vi "Hardware-ESTTL-Host.vi"() -> ()   [LabVIEW 2016]
uses:
  <vilib>/Powertrain Controls/Device Drivers/DCM/ESTTL/RT/Setup.ctl
  <vilib>/Powertrain Controls/Device Drivers/DCM/ESTTL/FPGA/Mode.ctl
  <vilib>/Powertrain Controls/Device Drivers/DCM/ESTTL/RT/Angle Control.ctl
  Shared/Typedefs/DiffIO-PWM-Settings.ctl
  Shared/Typedefs/DiffIO-PWM-Settings-Array.ctl
  Shared/DSI-Shared.lvlib
  <vilib>/Powertrain Controls/Device Drivers/DCM/ESTTL/FPGA/DCM - FPGA - ESTTL.lvlib
  <vilib>/Powertrain Controls/Device Drivers/DCM/ESTTL/RT/DCM - RT - ESTTL.lvlib
panel:
  in  "_Hidden":enum32{"Page 1"}(tab)
  in  "Setup":T1[](array[typedef])=[{"Mode"=enum."Off", "Polarity"=FALSE, "Frequency [Hz]"=0.0, "Duty Cycle [%]"=0.0, "TDC Offset [CAD]"=0.0, "Window Start [DBTDC]"=0.0, "Window End [DBTDC]"=0.0, "Angles"=[{"Enable"=FALSE, "Location [DBTDC]"=0.0, "Duration [s]"=0.0}, {"Enable"=FALSE, "Location [DBTDC]"=0.0, "Duration [s]"=0.0}, {"Enable"=FALSE, "Location [DBTDC]"=0.0, "Duration [s]"=0.0}, {"Enable"=FALSE, "Location [DBTDC]"=0.0, "Duration [s]"=0.0}], "Skip Fire"=FALSE, "Skip Fire Index"=0}, {"Mode"=enum."Off", "Polarity"=FALSE, "Frequency [Hz]"=0.0, "Duty Cycle [%]"=0.0, "TDC Offset [CAD]"=0.0, "Window Start [DBTDC]"=0.0, "Window End [DBTDC]"=0.0, "Angles"=[{"Enable"=FALSE, "Location [DBTDC]"=0.0, "Duration [s]"=0.0}, {"Enable"=FALSE, "Location [DBTDC]"=0.0, "Duration [s]"=0.0}, {"Enable"=FALSE, "Location [DBTDC]"=0.0, "Duration [s]"=0.0}, {"Enable"=FALSE, "Location [DBTDC]"=0.0, "Duration [s]"=0.0}], "Skip Fire"=FALSE, "Skip Fire Index"=0}, {"Mode"=enum."Off", "Polarity"=FALSE, "Frequency [Hz]"=0.0, "Duty Cycle [%]"=0.0, "TDC Offset [CAD]"=0.0, "Window Start [DBTDC]"=0.0, "Window End [DBTDC]"=0.0, "Angles"=[{"Enable"=FALSE, "Location [DBTDC]"=0.0, "Duration [s]"=0.0}, {"Enable"=FALSE, "Location [DBTDC]"=0.0, "Duration [s]"=0.0}, {"Enable"=FALSE, "Location [DBTDC]"=0.0, "Duration [s]"=0.0}, {"Enable"=FALSE, "Location [DBTDC]"=0.0, "Duration [s]"=0.0}], "Skip Fire"=FALSE, "Skip Fire Index"=0}, {"Mode"=enum."Off", "Polarity"=FALSE, "Frequency [Hz]"=0.0, "Duty Cycle [%]"=0.0, "TDC Offset [CAD]"=0.0, "Window Start [DBTDC]"=0.0, "Window End [DBTDC]"=0.0, "Angles"=[{"Enable"=FALSE, "Location [DBTDC]"=0.0, "Duration [s]"=0.0}, {"Enable"=FALSE, "Location [DBTDC]"=0.0, "Duration [s]"=0.0}, {"Enable"=FALSE, "Location [DBTDC]"=0.0, "Duration [s]"=0.0}, {"Enable"=FALSE, "Location [DBTDC]"=0.0, "Duration [s]"=0.0}], "Skip Fire"=FALSE, "Skip Fire Index"=0}, {"Mode"=enum."Off", "Polarity"=FALSE, "Frequency [Hz]"=0.0, "Duty Cycle [%]"=0.0, "TDC Offset [CAD]"=0.0, "Window Start [DBTDC]"=0.0, "Window End [DBTDC]"=0.0, "Angles"=[{"Enable"=FALSE, "Location [DBTDC]"=0.0, "Duration [s]"=0.0}, {"Enable"=FALSE, "Location [DBTDC]"=0.0, "Duration [s]"=0.0}, {"Enable"=FALSE, "Location [DBTDC]"=0.0, "Duration [s]"=0.0}, {"Enable"=FALSE, "Location [DBTDC]"=0.0, "Duration [s]"=0.0}], "Skip Fire"=FALSE, "Skip Fire Index"=0}, {"Mode"=enum."Off", "Polarity"=FALSE, "Frequency [Hz]"=0.0, "Duty Cycle [%]"=0.0, "TDC Offset [CAD]"=0.0, "Window Start [DBTDC]"=0.0, "Window End [DBTDC]"=0.0, "Angles"=[{"Enable"=FALSE, "Location [DBTDC]"=0.0, "Duration [s]"=0.0}, {"Enable"=FALSE, "Location [DBTDC]"=0.0, "Duration [s]"=0.0}, {"Enable"=FALSE, "Location [DBTDC]"=0.0, "Duration [s]"=0.0}, {"Enable"=FALSE, "Location [DBTDC]"=0.0, "Duration [s]"=0.0}], "Skip Fire"=FALSE, "Skip Fire Index"=0}, {"Mode"=enum."Off", "Polarity"=FALSE, "Frequency [Hz]"=0.0, "Duty Cycle [%]"=0.0, "TDC Offset [CAD]"=0.0, "Window Start [DBTDC]"=0.0, "Window End [DBTDC]"=0.0, "Angles"=[{"Enable"=FALSE, "Location [DBTDC]"=0.0, "Duration [s]"=0.0}, {"Enable"=FALSE, "Location [DBTDC]"=0.0, "Duration [s]"=0.0}, {"Enable"=FALSE, "Location [DBTDC]"=0.0, "Duration [s]"=0.0}, {"Enable"=FALSE, "Location [DBTDC]"=0.0, "Duration [s]"=0.0}], "Skip Fire"=FALSE, "Skip Fire Index"=0}, {"Mode"=enum."Off", "Polarity"=FALSE, "Frequency [Hz]"=0.0, "Duty Cycle [%]"=0.0, "TDC Offset [CAD]"=0.0, "Window Start [DBTDC]"=0.0, "Window End [DBTDC]"=0.0, "Angles"=[{"Enable"=FALSE, "Location [DBTDC]"=0.0, "Duration [s]"=0.0}, {"Enable"=FALSE, "Location [DBTDC]"=0.0, "Duration [s]"=0.0}, {"Enable"=FALSE, "Location [DBTDC]"=0.0, "Duration [s]"=0.0}, {"Enable"=FALSE, "Location [DBTDC]"=0.0, "Duration [s]"=0.0}], "Skip Fire"=FALSE, "Skip Fire Index"=0}] {"Skip Fire Index" max=7; "Angles"."Duration [s]" format="%#_3p"; "Frequency [Hz]" format="%#_3p"}
  in  "_Refresh":bool
  in  "AdaptMode":u32
  in  "ChannelNames":string[](array[string])
  in  "PWMSettings":T4=[{"PWM-TimingMode"=enum."Frequency", "PWM-Frequency"=0.0, "PWM-Period"=0.0, "PWM-ControlMode"=enum."Duty Cycle", "PWM-DutyCycle"=0.0, "PWM-PulseWidth"=0.0}, {"PWM-TimingMode"=enum."Frequency", "PWM-Frequency"=0.0, "PWM-Period"=0.0, "PWM-ControlMode"=enum."Duty Cycle", "PWM-DutyCycle"=0.0, "PWM-PulseWidth"=0.0}, {"PWM-TimingMode"=enum."Frequency", "PWM-Frequency"=0.0, "PWM-Period"=0.0, "PWM-ControlMode"=enum."Duty Cycle", "PWM-DutyCycle"=0.0, "PWM-PulseWidth"=0.0}, {"PWM-TimingMode"=enum."Frequency", "PWM-Frequency"=0.0, "PWM-Period"=0.0, "PWM-ControlMode"=enum."Duty Cycle", "PWM-DutyCycle"=0.0, "PWM-PulseWidth"=0.0}, {"PWM-TimingMode"=enum."Frequency", "PWM-Frequency"=0.0, "PWM-Period"=0.0, "PWM-ControlMode"=enum."Duty Cycle", "PWM-DutyCycle"=0.0, "PWM-PulseWidth"=0.0}, {"PWM-TimingMode"=enum."Frequency", "PWM-Frequency"=0.0, "PWM-Period"=0.0, "PWM-ControlMode"=enum."Duty Cycle", "PWM-DutyCycle"=0.0, "PWM-PulseWidth"=0.0}, {"PWM-TimingMode"=enum."Frequency", "PWM-Frequency"=0.0, "PWM-Period"=0.0, "PWM-ControlMode"=enum."Duty Cycle", "PWM-DutyCycle"=0.0, "PWM-PulseWidth"=0.0}, {"PWM-TimingMode"=enum."Frequency", "PWM-Frequency"=0.0, "PWM-Period"=0.0, "PWM-ControlMode"=enum."Duty Cycle", "PWM-DutyCycle"=0.0, "PWM-PulseWidth"=0.0}] caption="Advanced PWM Settings" {"PWM-Period" format="%#_2p"; "PWM-PulseWidth" format="%#_2p"; "PWM-DutyCycle" format="%#_2p"; "PWM-Frequency" format="%#_2p"}
  in  "_PWM Settings Element":T5 caption="Advanced PWM Settings" {"PWM-Period" format="%#_2p"; "PWM-PulseWidth" format="%#_2p"; "PWM-DutyCycle" format="%#_2p"; "PWM-Frequency" format="%#_2p"}
  in  "_Setup Tab":enum32{"Page 1"}(tab)
  in  "_SetupElement":T1={"Mode"=enum."Off", "Polarity"=FALSE, "Frequency [Hz]"=0.0, "Duty Cycle [%]"=0.0, "TDC Offset [CAD]"=0.0, "Window Start [DBTDC]"=0.0, "Window End [DBTDC]"=0.0, "Angles"=[{"Enable"=FALSE, "Location [DBTDC]"=0.0, "Duration [s]"=0.0}, {"Enable"=FALSE, "Location [DBTDC]"=0.0, "Duration [s]"=0.0}, {"Enable"=FALSE, "Location [DBTDC]"=0.0, "Duration [s]"=0.0}, {"Enable"=FALSE, "Location [DBTDC]"=0.0, "Duration [s]"=0.0}], "Skip Fire"=FALSE, "Skip Fire Index"=0} caption="Command Setup" {"Skip Fire Index" max=7; "Angles"."Duration [s]" format="%#_3p"; "Frequency [Hz]" format="%#_3p"}
  in  "_AdaptMode":bool caption="Adapt Mode"
  in  "_Channel Name":string caption="Name"
  in  "_ESTTL Channels":i32[](listbox) caption="ESTTL Channel Summary"
  # "Engine Synchronous TTL (ESTTL) Setup"
  # "Channel Settings"
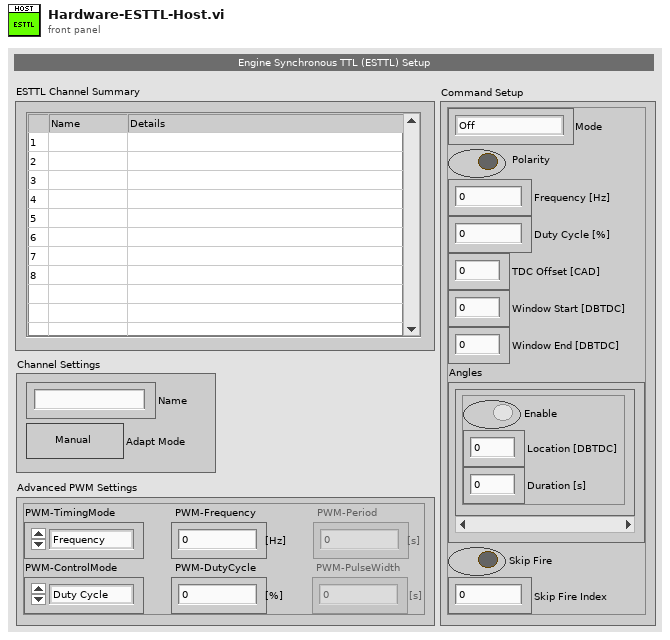
[diagram p1: front panel]
types:
  T1 = typedef "DCM - RT - ESTTL.lvlib/Setup.ctl" = cluster{"Mode":T2, "Polarity":bool, "Frequency [Hz]":sgl, "Duty Cycle [%]":sgl, "TDC Offset [CAD]":sgl, "Window Start [DBTDC]":sgl, "Window End [DBTDC]":sgl, "Angles":T3[], "Skip Fire":bool, "Skip Fire Index":u8}
  T2 = typedef "DCM - FPGA - ESTTL.lvlib/Mode.ctl" = enum8{"Off", "Pulse Width Modulation", "Engine Position Tracking"}
  T3 = typedef "DCM - RT - ESTTL.lvlib/Angle Control.ctl" = cluster{"Enable":bool, "Location [DBTDC]":sgl, "Duration [s]":sgl}
  T4 = typedef "DSI-Shared.lvlib/DiffIO-PWM-Settings-Array.ctl" = T5[]
  T5 = typedef "DSI-Shared.lvlib/DiffIO-PWM-Settings.ctl" = cluster{"PWM-TimingMode":enum32{"Frequency", "Period"}, "PWM-Frequency":sgl, "PWM-Period":sgl, "PWM-ControlMode":enum32{"Duty Cycle", "Pulsewidth"}, "PWM-DutyCycle":sgl, "PWM-PulseWidth":sgl}
  T6 = enum8{"Enabled", "Disabled", "Disabled and Grayed Out"}
  T7 = enum32{"Invalid", "Standard", "Closed", "Hidden", "Minimized", "Maximized"}
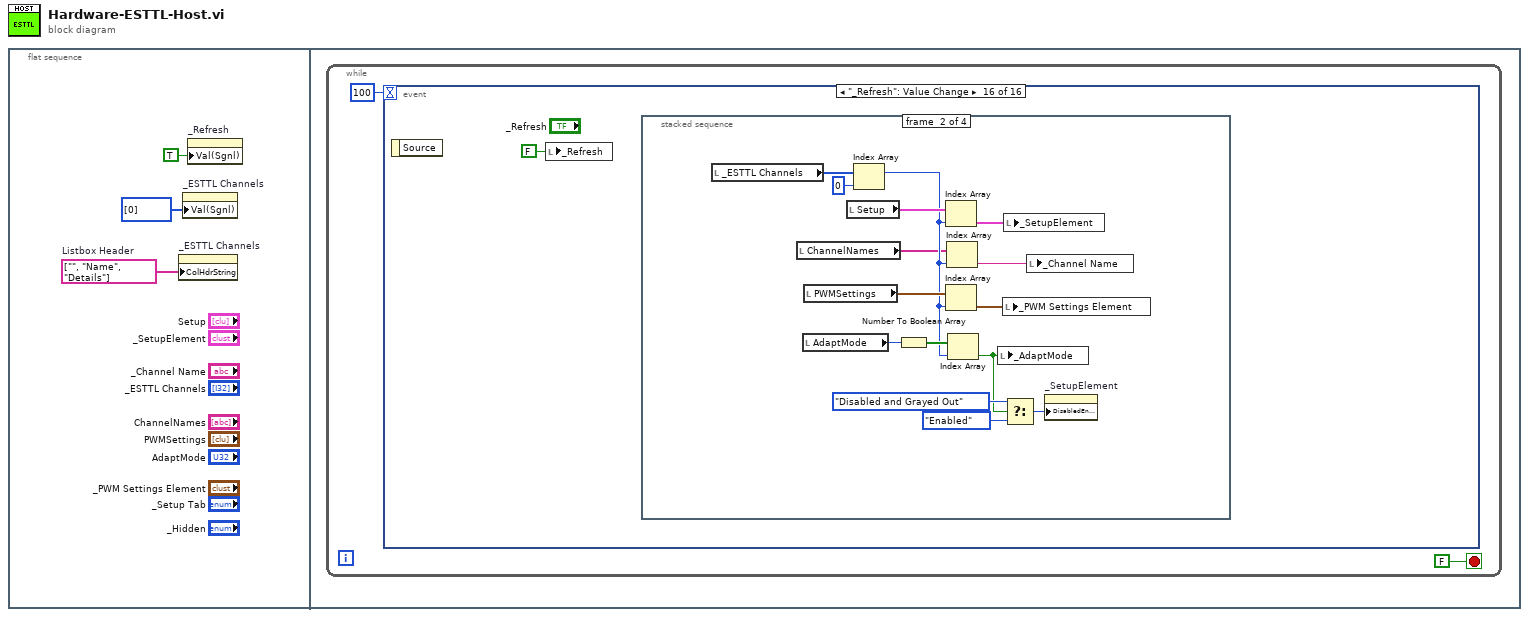
[diagram p0: block diagram]
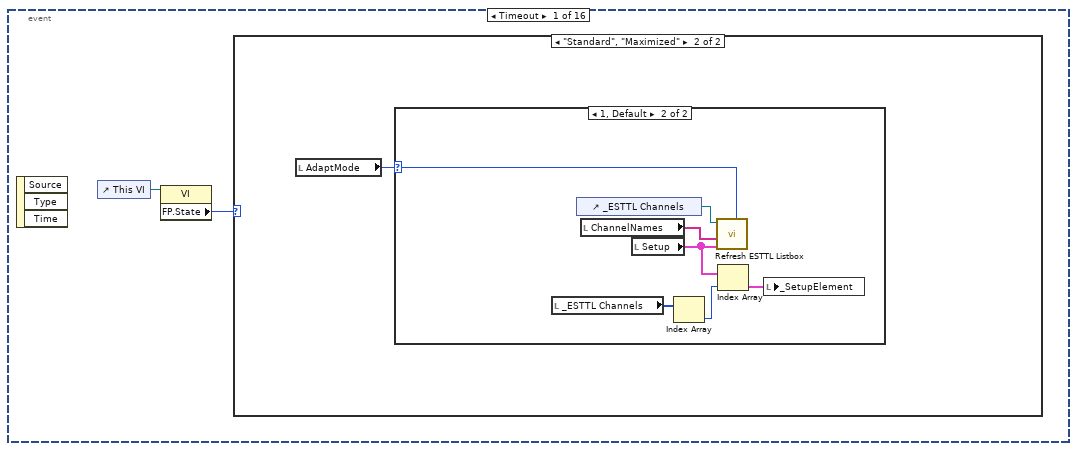
[diagram p2: hidden frame]
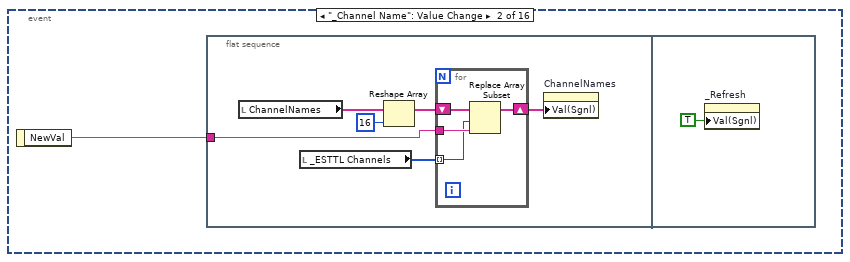
[diagram p5: hidden frame]
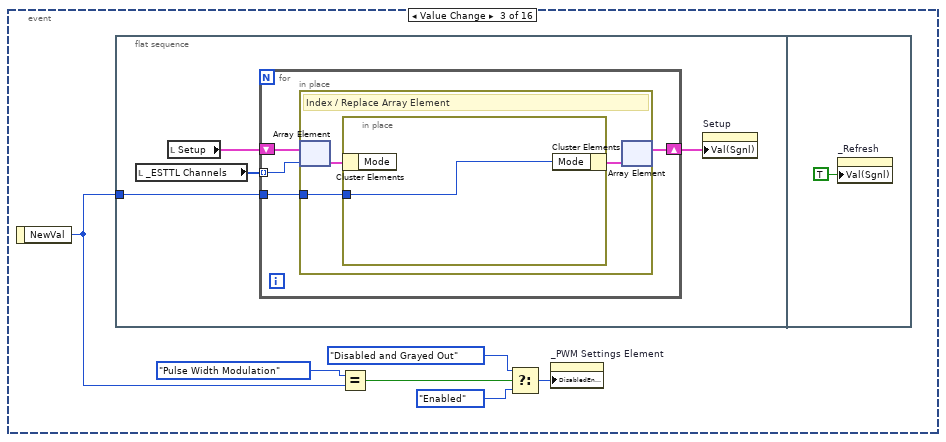
[diagram p6: hidden frame]
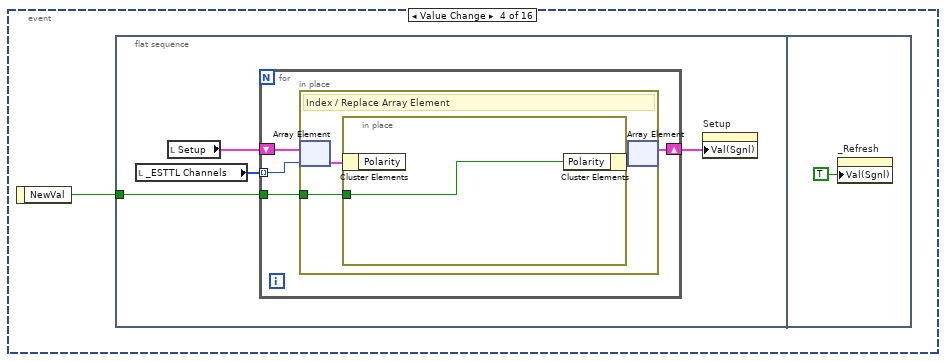
[diagram p7: hidden frame]
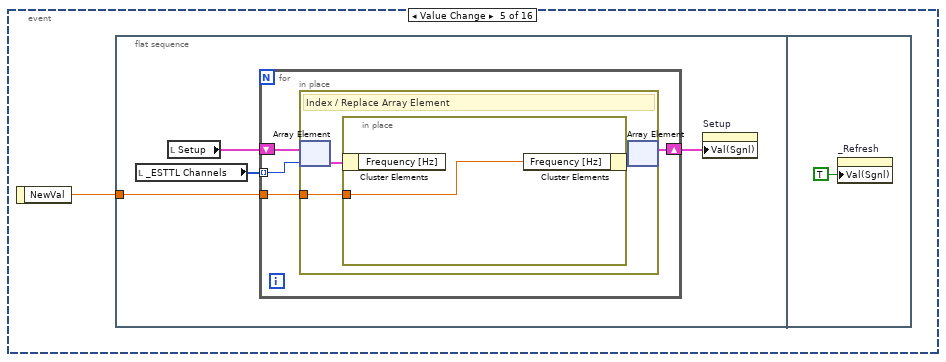
[diagram p8: hidden frame]
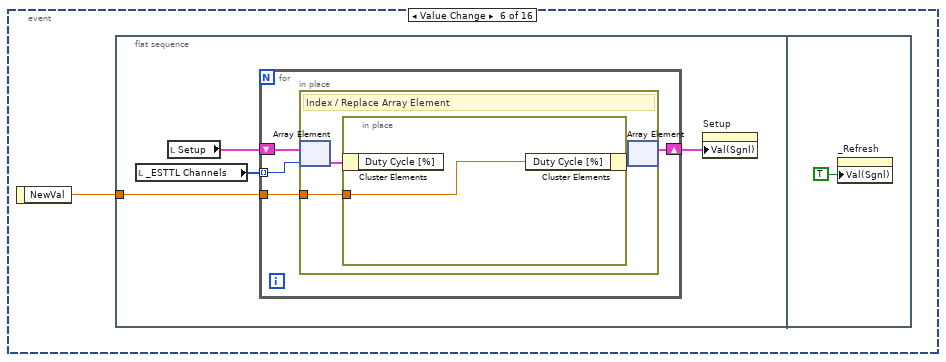
[diagram p9: hidden frame]
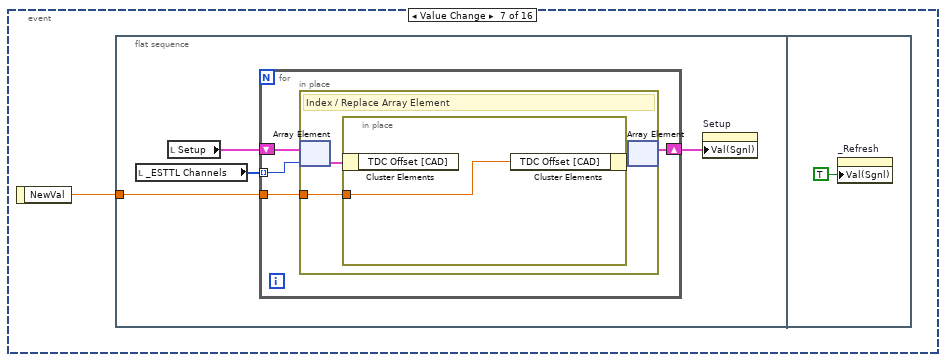
[diagram p10: hidden frame]
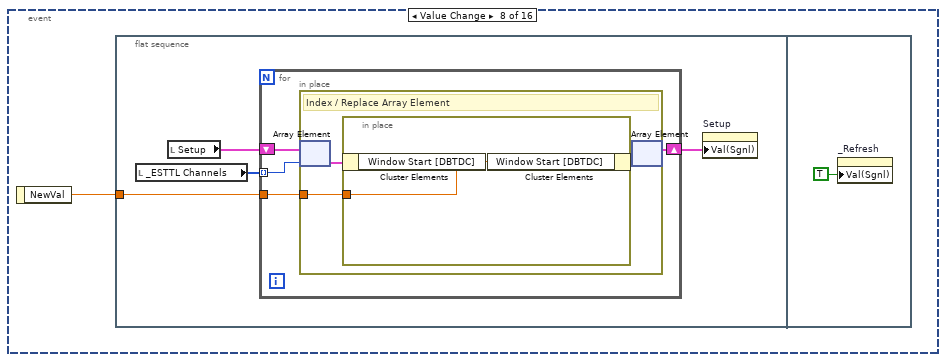
[diagram p11: hidden frame]
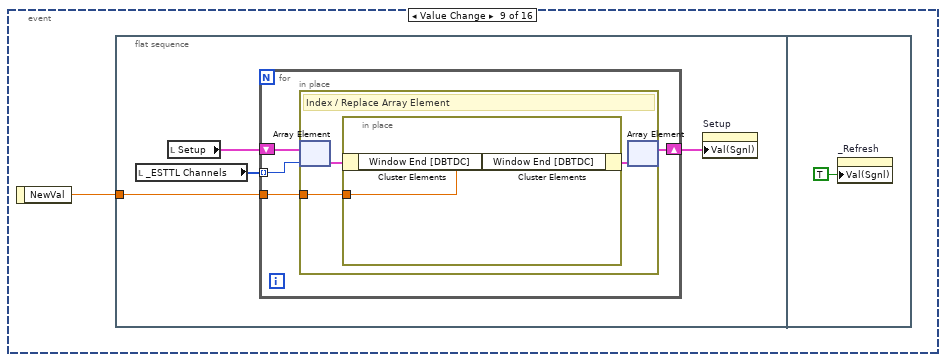
[diagram p12: hidden frame]
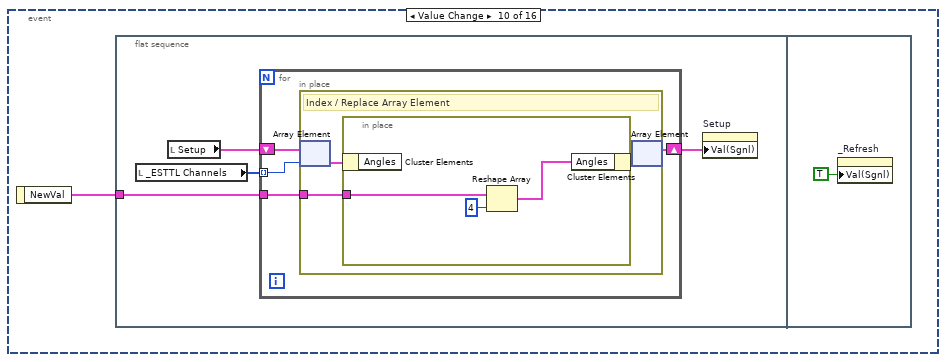
[diagram p13: hidden frame]
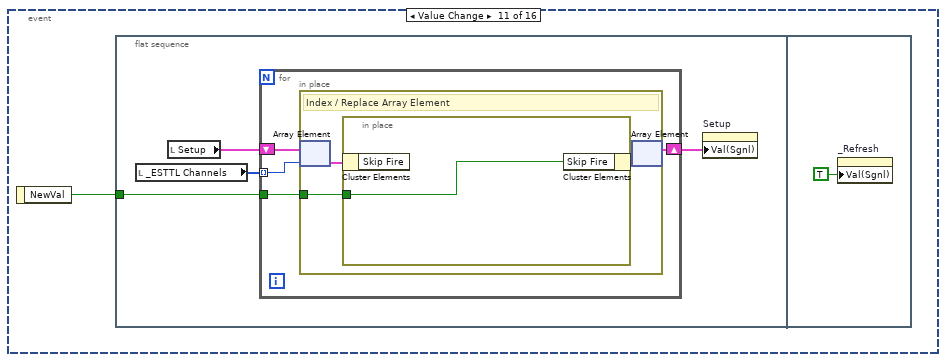
[diagram p14: hidden frame]
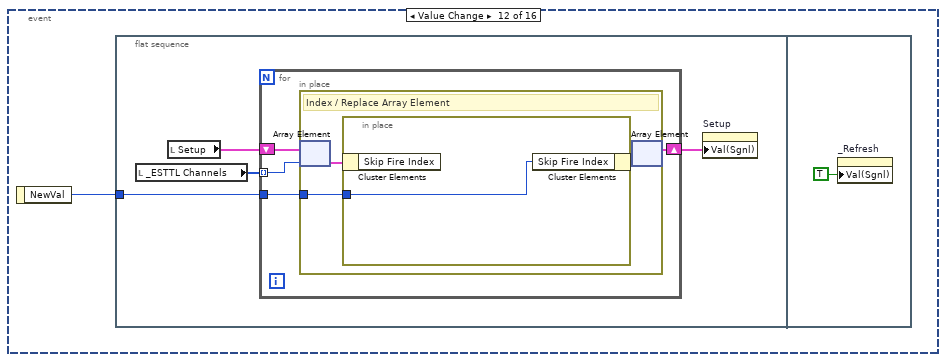
[diagram p15: hidden frame]
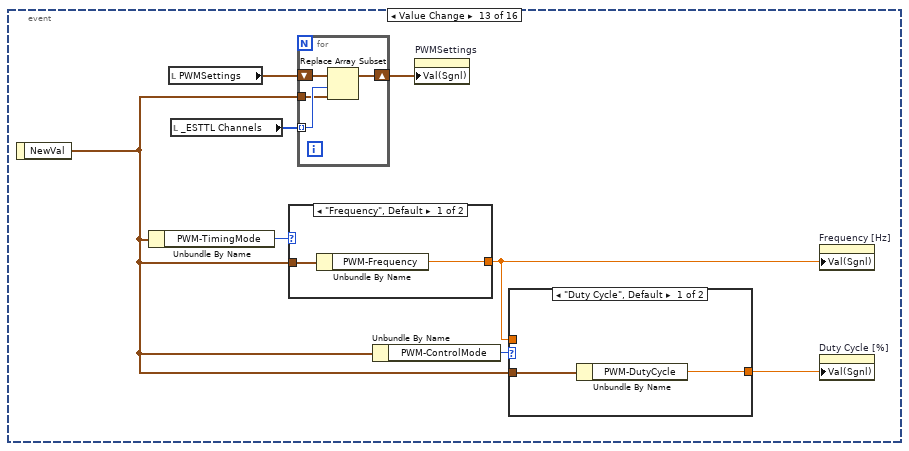
[diagram p16: hidden frame]
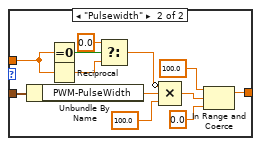
[diagram p17: hidden frame]
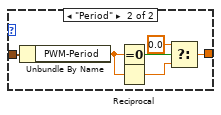
[diagram p18: hidden frame]
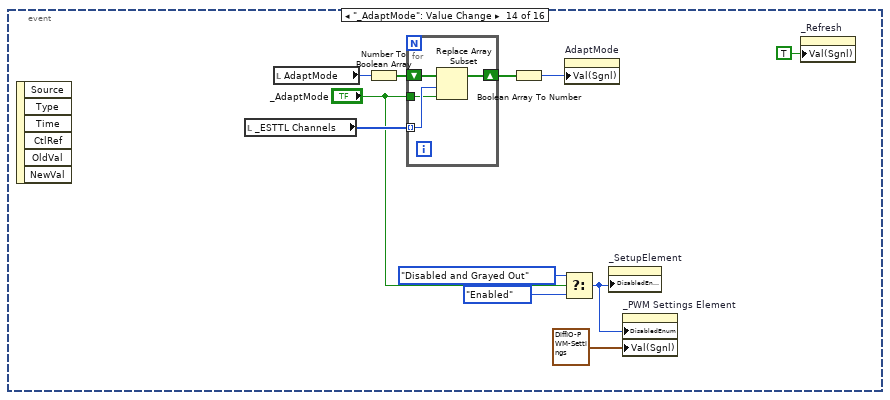
[diagram p19: hidden frame]
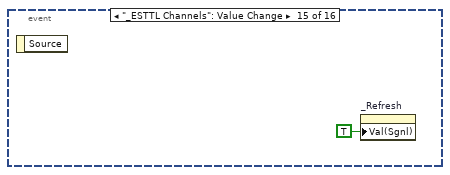
[diagram p20: hidden frame]
diagram:
  n1 = flat-sequence "Initialization code" {
    frame #0 {
      w3 = string[] ["", "Name", "Details"]  # Listbox Header
      n2 = property on="_ESTTL Channels" class="MCListbox (strict)"("ColHdrString"=w3) -> ()  [unwired: 2 in, 2 out]
      n3 = property on="_ESTTL Channels" class="MCListbox (strict)"("Val(Sgnl)"=i32[] [0] ("Value (Signaling)")) -> ()  [unwired: 2 in, 2 out]
      n4 = property on="_Refresh" class="Bool (strict)"("Val(Sgnl)"=TRUE ("Value (Signaling)")) -> ()  [unwired: 2 in, 2 out]
    }
    frame #1 {
      n5 = while {
        stop <- FALSE stop-if-true
        n6 = event shown="[15] \"_Refresh\": Value Change" {
          selector: _ -> [_ _ _ _ _ _ _ _ _ _ _ _ _ _ _ _]
          dyn-events: _ -> [_ _ _ _ _ _ _ _ _ _ _ _ _ _ _ _]
          timeout: 100 -> [_ _ _ _ _ _ _ _ _ _ _ _ _ _ _ _]
          event Timeout {
            n7 = event-data() -> ()  [unwired: 4 out]
            n8 = control-ref of="This VI"() -> (w7:refnum<vi>)
            n9 = property class="VI"(reference=w7) -> ("FP.State"=w6:T7)  [unwired: 1 in, 2 out]
            n10 = case shown="\"Standard\", \"Maximized\"" w6 {
              frame "Invalid", Default {
              }
              frame "Standard", "Maximized" {
                n11 = local read "AdaptMode"() -> (w8:u32)
                n12 = case shown="1, Default" w8 {
                  selector: w8 -> [_ w10]
                  frame 0 {
                  }
                  frame 1, Default {
                    n13 = local read "_ESTTL Channels"() -> (w15:i32[])
                    n14 = control-ref of="_ESTTL Channels"() -> (w12:refnum<vi>)
                    n15 = local read "ChannelNames"() -> (w9:string[])
                    n16 = local read "Setup"() -> (w11:T1[])
                    n17 = Index Array(array=w15) -> (element=w14:i32)  [unwired: 1 in]
                    n18 = call "Refresh ESTTL Listbox.vi"("AdaptMode"=w10, "Setup"=w11, "Names"=w9, "_ESTTL Channels"=w12) -> ()  [unwired: 8 in]
                    n19 = Index Array(array=w11, index=w14) -> (element=w13:T1)
                    n20 = local write "_SetupElement"(w13) -> ()
                  }
                }
              }
            }
          }
          event "_Channel Name": Value Change {
            n21 = event-data() -> ("NewVal"=w16:string)  [unwired: 1 out]
            n22 = flat-sequence {
              tunnel: w16 -> [w20]
              frame #0 {
                n23 = local read "ChannelNames"() -> (w18:string[])
                n24 = local read "_ESTTL Channels"() -> (w19:i32[])
                n25 = Reshape Array(w18, 16 ("dimension size")) -> (w22:string[])
                n26 = for {
                  tunnel: w20 -> [w24]
                  shift-right: [w26] -> w17
                  shift-left: w22 -> [w25]
                  tunnel: w19 -> [w23] mode=indexing
                  n27 = Replace Array Subset(array=w25, new element=w24, index=w23) -> (w26:string[])
                }
                n28 = property on="ChannelNames" class="Arr (strict)"("Val(Sgnl)"=w17) -> ()  [unwired: 2 in, 2 out]
              }
              frame #1 {
                n29 = property on="_Refresh" class="Bool (strict)"("Val(Sgnl)"=TRUE ("Value (Signaling)")) -> ()  [unwired: 2 in, 2 out]
              }
            }
          }
          event Value Change {
            n30 = event-data() -> ("NewVal"=w29:T2)  [unwired: 1 out]
            n31 = flat-sequence {
              tunnel: w29 -> [w36]
              frame #0 {
                n32 = local read "_ESTTL Channels"() -> (w37:i32[])
                n33 = local read "Setup"() -> (w35:T1[])
                n34 = for {
                  tunnel: w37 -> [w40] mode=indexing
                  shift-right: [w39] -> w34
                  shift-left: w35 -> [w41]
                  tunnel: w36 -> [w38]
                  n35 = in-place {
                    in-place-border: w38 -> [w42]
                    # "Index / Replace Array Element"
                    n36 = in-place-array #1(w41, w40) -> (w44:T1)
                    n37 = in-place {
                      in-place-border: w42 -> [w45]
                      n38 = in-place-cluster #2(w44) -> ()  [unwired: 1 out]
                      n39 = in-place-cluster #2("Mode"=w45) -> (w43:T1)
                    }
                    n40 = in-place-array #1(w43) -> (w39:T1[])  [unwired: 1 out]
                  }
                }
                n41 = property on="Setup" class="Arr (strict)"("Val(Sgnl)"=w34) -> ()  [unwired: 2 in, 2 out]
              }
              frame #1 {
                n42 = property on="_Refresh" class="Bool (strict)"("Val(Sgnl)"=TRUE ("Value (Signaling)")) -> ()  [unwired: 2 in, 2 out]
              }
            }
            n43 = Equal?(x=Mode."Pulse Width Modulation" ("NewVal"), y=w29) -> (x = y?=w31:bool)
            n44 = Select(t=T6."Disabled and Grayed Out" ("Disabled"), s=w31, f=T6."Enabled" ("Disabled")) -> (s? t:f=w30:T6)
            n45 = property on="_PWM Settings Element" class="Clust (strict)"("DisabledEnum"=w30) -> ()  [unwired: 2 in, 2 out]
          }
          event Value Change {
            n46 = event-data() -> ("NewVal"=w47:bool)  [unwired: 1 out]
            n47 = flat-sequence {
              tunnel: w47 -> [w50]
              frame #0 {
                n48 = local read "_ESTTL Channels"() -> (w51:i32[])
                n49 = local read "Setup"() -> (w49:T1[])
                n50 = for {
                  tunnel: w51 -> [w54] mode=indexing
                  shift-right: [w53] -> w48
                  shift-left: w49 -> [w55]
                  tunnel: w50 -> [w52]
                  n51 = in-place {
                    in-place-border: w52 -> [w56]
                    # "Index / Replace Array Element"
                    n52 = in-place-array #3(w55, w54) -> (w58:T1)
                    n53 = in-place {
                      in-place-border: w56 -> [w59]
                      n54 = in-place-cluster #4(w58) -> ()  [unwired: 1 out]
                      n55 = in-place-cluster #4("Polarity"=w59) -> (w57:T1)
                    }
                    n56 = in-place-array #3(w57) -> (w53:T1[])  [unwired: 1 out]
                  }
                }
                n57 = property on="Setup" class="Arr (strict)"("Val(Sgnl)"=w48) -> ()  [unwired: 2 in, 2 out]
              }
              frame #1 {
                n58 = property on="_Refresh" class="Bool (strict)"("Val(Sgnl)"=TRUE ("Value (Signaling)")) -> ()  [unwired: 2 in, 2 out]
              }
            }
          }
          event Value Change {
            n59 = event-data() -> ("NewVal"=w61:sgl)  [unwired: 1 out]
            n60 = flat-sequence {
              tunnel: w61 -> [w64]
              frame #0 {
                n61 = local read "_ESTTL Channels"() -> (w65:i32[])
                n62 = local read "Setup"() -> (w63:T1[])
                n63 = for {
                  tunnel: w65 -> [w68] mode=indexing
                  shift-right: [w67] -> w62
                  shift-left: w63 -> [w69]
                  tunnel: w64 -> [w66]
                  n64 = in-place {
                    in-place-border: w66 -> [w70]
                    # "Index / Replace Array Element"
                    n65 = in-place-array #5(w69, w68) -> (w72:T1)
                    n66 = in-place {
                      in-place-border: w70 -> [w73]
                      n67 = in-place-cluster #6(w72) -> ()  [unwired: 1 out]
                      n68 = in-place-cluster #6("Frequency [Hz]"=w73) -> (w71:T1)
                    }
                    n69 = in-place-array #5(w71) -> (w67:T1[])  [unwired: 1 out]
                  }
                }
                n70 = property on="Setup" class="Arr (strict)"("Val(Sgnl)"=w62) -> ()  [unwired: 2 in, 2 out]
              }
              frame #1 {
                n71 = property on="_Refresh" class="Bool (strict)"("Val(Sgnl)"=TRUE ("Value (Signaling)")) -> ()  [unwired: 2 in, 2 out]
              }
            }
          }
          event Value Change {
            n72 = event-data() -> ("NewVal"=w75:sgl)  [unwired: 1 out]
            n73 = flat-sequence {
              tunnel: w75 -> [w78]
              frame #0 {
                n74 = local read "_ESTTL Channels"() -> (w79:i32[])
                n75 = local read "Setup"() -> (w77:T1[])
                n76 = for {
                  tunnel: w79 -> [w82] mode=indexing
                  shift-right: [w81] -> w76
                  shift-left: w77 -> [w83]
                  tunnel: w78 -> [w80]
                  n77 = in-place {
                    in-place-border: w80 -> [w84]
                    # "Index / Replace Array Element"
                    n78 = in-place-array #7(w83, w82) -> (w86:T1)
                    n79 = in-place {
                      in-place-border: w84 -> [w87]
                      n80 = in-place-cluster #8(w86) -> ()  [unwired: 1 out]
                      n81 = in-place-cluster #8("Duty Cycle [%]"=w87) -> (w85:T1)
                    }
                    n82 = in-place-array #7(w85) -> (w81:T1[])  [unwired: 1 out]
                  }
                }
                n83 = property on="Setup" class="Arr (strict)"("Val(Sgnl)"=w76) -> ()  [unwired: 2 in, 2 out]
              }
              frame #1 {
                n84 = property on="_Refresh" class="Bool (strict)"("Val(Sgnl)"=TRUE ("Value (Signaling)")) -> ()  [unwired: 2 in, 2 out]
              }
            }
          }
          event Value Change {
            n85 = event-data() -> ("NewVal"=w89:sgl)  [unwired: 1 out]
            n86 = flat-sequence {
              tunnel: w89 -> [w92]
              frame #0 {
                n87 = local read "_ESTTL Channels"() -> (w93:i32[])
                n88 = local read "Setup"() -> (w91:T1[])
                n89 = for {
                  tunnel: w93 -> [w96] mode=indexing
                  shift-right: [w95] -> w90
                  shift-left: w91 -> [w97]
                  tunnel: w92 -> [w94]
                  n90 = in-place {
                    in-place-border: w94 -> [w98]
                    # "Index / Replace Array Element"
                    n91 = in-place-array #9(w97, w96) -> (w100:T1)
                    n92 = in-place {
                      in-place-border: w98 -> [w101]
                      n93 = in-place-cluster #10(w100) -> ()  [unwired: 1 out]
                      n94 = in-place-cluster #10("TDC Offset [CAD]"=w101) -> (w99:T1)
                    }
                    n95 = in-place-array #9(w99) -> (w95:T1[])  [unwired: 1 out]
                  }
                }
                n96 = property on="Setup" class="Arr (strict)"("Val(Sgnl)"=w90) -> ()  [unwired: 2 in, 2 out]
              }
              frame #1 {
                n97 = property on="_Refresh" class="Bool (strict)"("Val(Sgnl)"=TRUE ("Value (Signaling)")) -> ()  [unwired: 2 in, 2 out]
              }
            }
          }
          event Value Change {
            n98 = event-data() -> ("NewVal"=w103:sgl)  [unwired: 1 out]
            n99 = flat-sequence {
              tunnel: w103 -> [w106]
              frame #0 {
                n100 = local read "_ESTTL Channels"() -> (w107:i32[])
                n101 = local read "Setup"() -> (w105:T1[])
                n102 = for {
                  tunnel: w107 -> [w110] mode=indexing
                  shift-right: [w109] -> w104
                  shift-left: w105 -> [w111]
                  tunnel: w106 -> [w108]
                  n103 = in-place {
                    in-place-border: w108 -> [w112]
                    # "Index / Replace Array Element"
                    n104 = in-place-array #11(w111, w110) -> (w114:T1)
                    n105 = in-place {
                      in-place-border: w112 -> [w115]
                      n106 = in-place-cluster #12(w114) -> ()  [unwired: 1 out]
                      n107 = in-place-cluster #12("Window Start [DBTDC]"=w115) -> (w113:T1)
                    }
                    n108 = in-place-array #11(w113) -> (w109:T1[])  [unwired: 1 out]
                  }
                }
                n109 = property on="Setup" class="Arr (strict)"("Val(Sgnl)"=w104) -> ()  [unwired: 2 in, 2 out]
              }
              frame #1 {
                n110 = property on="_Refresh" class="Bool (strict)"("Val(Sgnl)"=TRUE ("Value (Signaling)")) -> ()  [unwired: 2 in, 2 out]
              }
            }
          }
          event Value Change {
            n111 = event-data() -> ("NewVal"=w117:sgl)  [unwired: 1 out]
            n112 = flat-sequence {
              tunnel: w117 -> [w120]
              frame #0 {
                n113 = local read "_ESTTL Channels"() -> (w121:i32[])
                n114 = local read "Setup"() -> (w119:T1[])
                n115 = for {
                  tunnel: w121 -> [w124] mode=indexing
                  shift-right: [w123] -> w118
                  shift-left: w119 -> [w125]
                  tunnel: w120 -> [w122]
                  n116 = in-place {
                    in-place-border: w122 -> [w126]
                    # "Index / Replace Array Element"
                    n117 = in-place-array #13(w125, w124) -> (w128:T1)
                    n118 = in-place {
                      in-place-border: w126 -> [w129]
                      n119 = in-place-cluster #14(w128) -> ()  [unwired: 1 out]
                      n120 = in-place-cluster #14("Window End [DBTDC]"=w129) -> (w127:T1)
                    }
                    n121 = in-place-array #13(w127) -> (w123:T1[])  [unwired: 1 out]
                  }
                }
                n122 = property on="Setup" class="Arr (strict)"("Val(Sgnl)"=w118) -> ()  [unwired: 2 in, 2 out]
              }
              frame #1 {
                n123 = property on="_Refresh" class="Bool (strict)"("Val(Sgnl)"=TRUE ("Value (Signaling)")) -> ()  [unwired: 2 in, 2 out]
              }
            }
          }
          event Value Change {
            n124 = event-data() -> ("NewVal"=w131:T3[])  [unwired: 1 out]
            n125 = flat-sequence {
              tunnel: w131 -> [w134]
              frame #0 {
                n126 = local read "_ESTTL Channels"() -> (w135:i32[])
                n127 = local read "Setup"() -> (w133:T1[])
                n128 = for {
                  tunnel: w135 -> [w138] mode=indexing
                  shift-right: [w137] -> w132
                  shift-left: w133 -> [w139]
                  tunnel: w134 -> [w136]
                  n129 = in-place {
                    in-place-border: w136 -> [w140]
                    # "Index / Replace Array Element"
                    n130 = in-place-array #15(w139, w138) -> (w142:T1)
                    n131 = in-place {
                      in-place-border: w140 -> [w144]
                      n132 = in-place-cluster #16(w142) -> ()  [unwired: 1 out]
                      n133 = Reshape Array(w144, 4 ("dimension size")) -> (w143:T3[])
                      n134 = in-place-cluster #16("Angles"=w143) -> (w141:T1)
                    }
                    n135 = in-place-array #15(w141) -> (w137:T1[])  [unwired: 1 out]
                  }
                }
                n136 = property on="Setup" class="Arr (strict)"("Val(Sgnl)"=w132) -> ()  [unwired: 2 in, 2 out]
              }
              frame #1 {
                n137 = property on="_Refresh" class="Bool (strict)"("Val(Sgnl)"=TRUE ("Value (Signaling)")) -> ()  [unwired: 2 in, 2 out]
              }
            }
          }
          event Value Change {
            n138 = event-data() -> ("NewVal"=w147:bool)  [unwired: 1 out]
            n139 = flat-sequence {
              tunnel: w147 -> [w150]
              frame #0 {
                n140 = local read "_ESTTL Channels"() -> (w151:i32[])
                n141 = local read "Setup"() -> (w149:T1[])
                n142 = for {
                  tunnel: w151 -> [w154] mode=indexing
                  shift-right: [w153] -> w148
                  shift-left: w149 -> [w155]
                  tunnel: w150 -> [w152]
                  n143 = in-place {
                    in-place-border: w152 -> [w156]
                    # "Index / Replace Array Element"
                    n144 = in-place-array #17(w155, w154) -> (w158:T1)
                    n145 = in-place {
                      in-place-border: w156 -> [w159]
                      n146 = in-place-cluster #18(w158) -> ()  [unwired: 1 out]
                      n147 = in-place-cluster #18("Skip Fire"=w159) -> (w157:T1)
                    }
                    n148 = in-place-array #17(w157) -> (w153:T1[])  [unwired: 1 out]
                  }
                }
                n149 = property on="Setup" class="Arr (strict)"("Val(Sgnl)"=w148) -> ()  [unwired: 2 in, 2 out]
              }
              frame #1 {
                n150 = property on="_Refresh" class="Bool (strict)"("Val(Sgnl)"=TRUE ("Value (Signaling)")) -> ()  [unwired: 2 in, 2 out]
              }
            }
          }
          event Value Change {
            n151 = event-data() -> ("NewVal"=w161:u8)  [unwired: 1 out]
            n152 = flat-sequence {
              tunnel: w161 -> [w164]
              frame #0 {
                n153 = local read "_ESTTL Channels"() -> (w165:i32[])
                n154 = local read "Setup"() -> (w163:T1[])
                n155 = for {
                  tunnel: w165 -> [w168] mode=indexing
                  shift-right: [w167] -> w162
                  shift-left: w163 -> [w169]
                  tunnel: w164 -> [w166]
                  n156 = in-place {
                    in-place-border: w166 -> [w170]
                    # "Index / Replace Array Element"
                    n157 = in-place-array #19(w169, w168) -> (w172:T1)
                    n158 = in-place {
                      in-place-border: w170 -> [w173]
                      n159 = in-place-cluster #20(w172) -> ()  [unwired: 1 out]
                      n160 = in-place-cluster #20("Skip Fire Index"=w173) -> (w171:T1)
                    }
                    n161 = in-place-array #19(w171) -> (w167:T1[])  [unwired: 1 out]
                  }
                }
                n162 = property on="Setup" class="Arr (strict)"("Val(Sgnl)"=w162) -> ()  [unwired: 2 in, 2 out]
              }
              frame #1 {
                n163 = property on="_Refresh" class="Bool (strict)"("Val(Sgnl)"=TRUE ("Value (Signaling)")) -> ()  [unwired: 2 in, 2 out]
              }
            }
          }
          event Value Change {
            n164 = event-data() -> ("NewVal"=w177:T5)  [unwired: 1 out]
            n165 = Unbundle By Name(w177) -> ("PWM-TimingMode"=w181:enum32{"Frequency", "Period"})
            n166 = local read "PWMSettings"() -> (w180:T4)
            n167 = local read "_ESTTL Channels"() -> (w178:i32[])
            n168 = case shown="\"Frequency\", Default" w181 {
              tunnel: w177 -> [w202 w208]
              tunnel: [w201 w205] -> w176
              frame "Frequency", Default {
                n169 = Unbundle By Name(w202) -> ("PWM-Frequency"=w201:sgl)
              }
              frame "Period" {
                n170 = Unbundle By Name(w208) -> ("PWM-Period"=w203:sgl)
                n171 = Equal To 0?(x=w203) -> (x = 0?=w206:bool)
                n172 = Reciprocal(x=w203) -> (1/x=w207:sgl)
                n173 = Select(t=sgl 0.0, s=w206, f=w207) -> (s? t:f=w205:sgl)
              }
            }
            n174 = for {
              shift-right: [w185] -> w179
              shift-left: w180 -> [w184]
              tunnel: w178 -> [w186] mode=indexing
              tunnel: w177 -> [w183]
              n175 = Replace Array Subset(array=w184, new element=w183, index=w186) -> (w185:T4)
            }
            n176 = Unbundle By Name(w177) -> ("PWM-ControlMode"=w182:enum32{"Duty Cycle", "Pulsewidth"})
            n177 = property on="PWMSettings" class="Arr (strict)"("Val(Sgnl)"=w179) -> ()  [unwired: 2 in, 2 out]
            n178 = case shown="\"Duty Cycle\", Default" w182 {
              tunnel: w177 -> [w188 w200]
              tunnel: [w187 w190] -> w175
              tunnel: w176 -> [_ w194]
              frame "Duty Cycle", Default {
                n179 = Unbundle By Name(w188) -> ("PWM-DutyCycle"=w187:sgl)
              }
              frame "Pulsewidth" {
                n180 = Unbundle By Name(w200) -> ("PWM-PulseWidth"=w199:sgl)
                n181 = Equal To 0?(x=w194) -> (x = 0?=w197:bool)
                n182 = Reciprocal(x=w194) -> (1/x=w198:sgl)
                n183 = Select(t=sgl 0.0, s=w197, f=w198) -> (s? t:f=w195:sgl)
                n184 = Compound Arithmetic op=MULTIPLY(invert w195, w199, sgl 100.0 ("value")) -> (w193:sgl)
                n185 = In Range and Coerce(upper limit=sgl 100.0, x=w193, lower limit=sgl 0.0 ("upper limit")) -> (coerced(x)=w190:sgl)  [unwired: 1 out]
              }
            }
            n186 = property on="Frequency [Hz]" class="DigNum (strict)"("Val(Sgnl)"=w176) -> ()  [unwired: 2 in, 2 out]
            n187 = property on="Duty Cycle [%]" class="DigNum (strict)"("Val(Sgnl)"=w175) -> ()  [unwired: 2 in, 2 out]
          }
          event "_AdaptMode": Value Change {
            n188 = event-data() -> ()  [unwired: 7 out]
            n189 = local read "_ESTTL Channels"() -> (w211:i32[])
            n190 = local read "AdaptMode"() -> (w219:u32)
            n191 = Number To Boolean Array(number=w219) -> (Boolean array=w213:bool[])
            n192 = for {
              shift-right: [w222] -> w212
              shift-left: w213 -> [w221]
              tunnel: w211 -> [w223] mode=indexing
              tunnel: "_AdaptMode" -> [w220]
              n193 = Replace Array Subset(array=w221, new element=w220, index=w223) -> (w222:bool[])
            }
            n194 = Boolean Array To Number(Boolean array=w212) -> (number=w218:u32)
            n195 = Select(t=T6."Disabled and Grayed Out" ("Disabled"), s="_AdaptMode", f=T6."Enabled" ("Disabled")) -> (s? t:f=w214:T6)
            n196 = property on="AdaptMode" class="DigNum (strict)"("Val(Sgnl)"=w218) -> ()  [unwired: 2 in, 2 out]
            n197 = property on="_SetupElement" class="Clust (strict)"("DisabledEnum"=w214) -> ()  [unwired: 2 in, 2 out]
            n198 = property on="_PWM Settings Element" class="Clust (strict)"("DisabledEnum"=w214, "Val(Sgnl)"=T5 {"PWM-TimingMode"=enum."Frequency", "PWM-Frequency"=0.0, "PWM-Period"=0.0, "PWM-ControlMode"=enum."Duty Cycle", "PWM-DutyCycle"=0.0, "PWM-PulseWidth"=0.0} ("Value (Signaling)")) -> ()  [unwired: 2 in, 2 out]
            n199 = property on="_Refresh" class="Bool (strict)"("Val(Sgnl)"=TRUE ("Value (Signaling)")) -> ()  [unwired: 2 in, 2 out]
          }
          event "_ESTTL Channels": Value Change {
            n200 = event-data() -> ()  [unwired: 2 out]
            n201 = property on="_Refresh" class="Bool (strict)"("Val(Sgnl)"=TRUE ("Value (Signaling)")) -> ()  [unwired: 2 in, 2 out]
          }
          event "_Refresh": Value Change {
            n202 = event-data() -> ()  [unwired: 2 out]
            n203 = local write "_Refresh"(FALSE ("_Refresh")) -> ()
            n204 = stacked-sequence {
              frame #0 {
                n205 = call <vilib>:"Set Busy.vi"() -> ()  [unwired: 10 in, 2 out]
                n206 = Wait (ms)(milliseconds to wait=u32 100) -> ()  [unwired: 1 out]
              }
              frame #1 {
                n207 = local read "_ESTTL Channels"() -> (w231:i32[])
                n208 = local read "ChannelNames"() -> (w227:string[])
                n209 = local read "AdaptMode"() -> (w238:u32)
                n210 = local read "PWMSettings"() -> (w230:T4)
                n211 = local read "Setup"() -> (w241:T1[])
                n212 = Index Array(array=w231, index=0) -> (element=w228:i32)
                n213 = Number To Boolean Array(number=w238) -> (Boolean array=w237:bool[])
                n214 = Index Array(array=w241, index=w228) -> (element=w240:T1)
                n215 = Index Array(array=w230, index=w228) -> (element=w232:T5)
                n216 = Index Array(array=w227, index=w228) -> (element=w239:string)
                n217 = Index Array(array=w237, index=w228) -> (element=w234:bool)
                n218 = local write "_AdaptMode"(w234) -> ()
                n219 = local write "_PWM Settings Element"(w232) -> ()
                n220 = local write "_SetupElement"(w240) -> ()
                n221 = Select(t=T6."Disabled and Grayed Out" ("Disabled"), s=w234, f=T6."Enabled" ("Disabled")) -> (s? t:f=w233:T6)
                n222 = local write "_Channel Name"(w239) -> ()
                n223 = property on="_SetupElement" class="Clust (strict)"("DisabledEnum"=w233) -> ()  [unwired: 2 in, 2 out]
              }
              frame #2 {
                n224 = control-ref of="_SetupElement"() -> (w244:refnum<vi>)
                n225 = control-ref of="_ESTTL Channels"() -> (w246:refnum<vi>)
                n226 = local read "ChannelNames"() -> (w242:string[])
                n227 = local read "_SetupElement"() -> (w243:T1)
                n228 = local read "_AdaptMode"() -> (w245:bool)
                n229 = local read "AdaptMode"() -> (w248:u32)
                n230 = local read "Setup"() -> (w249:T1[])
                n231 = control-ref of="_PWM Settings Element"() -> (w247:refnum<vi>)
                n232 = call "ESTTL Command Disable.vi"("ESTTL Setup"=w244) -> ()  [unwired: 11 in]
                n233 = call "ESTTL PWM Disable.vi"("Adapting?"=w245, "_SetupElement"=w243, "Cluster in"=w247) -> ()  [unwired: 9 in]
                n234 = call "Refresh ESTTL Listbox.vi"("AdaptMode"=w248, "Setup"=w249, "Names"=w242, "_ESTTL Channels"=w246) -> ()  [unwired: 8 in]
              }
              frame #3 {
                n235 = call <vilib>:"Unset Busy.vi"() -> ()  [unwired: 11 in, 1 out]
              }
            }
          }
        }
      }
    }
  }
